vi "Constructor.vi"(8 "error in":errorcluster, 9 "Value":i64, 10 "Name":string, 11 "Integer in":refnum<class "Integer.lvclass">) -> (0 "error out":errorcluster, 3 "Integer out":refnum<class "Integer.lvclass">)   [LabVIEW 2021, in "ProligentXMLGenerator.lvlib" / "Integer.lvclass"]
uses:
  Integer.lvclass
  Integer.lvclass/Integer.ctl
  Attribute/Attribute.lvclass
  C:/Projects/proligent-xml-generator-labview/src/ProligentXMLGenerator/Base/Attribute/Attribute.lvclass
  C:/Projects/proligent-xml-generator-labview/src/ProligentXMLGenerator/Base/Integer/Integer.lvclass
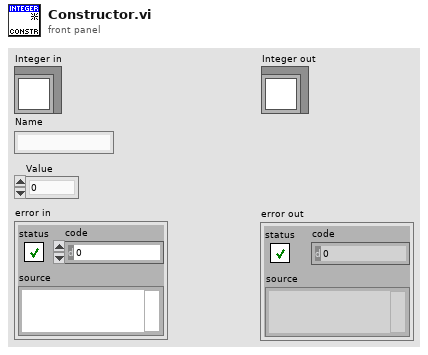
[diagram p1: front panel]
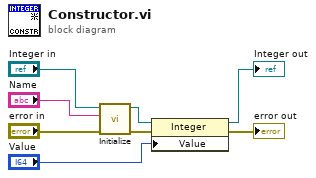
[diagram p0: block diagram]
diagram:
  n1 = call "Initialize.vi"("error in"="error in", "Name"="Name", "Attribute in"="Integer in") -> ("error out"=w4:errorcluster, "Attribute out"=w3:refnum<class "Integer.lvclass">)  [unwired: 7 in]
  n2 = property on="Property Node" class="Integer"(reference=w3, error in=w4, "Value"="Value") -> (reference out=→"Integer out":refnum<class "Integer.lvclass">, error out=→"error out":errorcluster)
